vi "Read Control Loop Response Power Analysis (Phase).vi"(8 "error in (no error)":errorcluster, 11 "VISA resource name":refnum<visa-resource-name>) -> (0 "error out":errorcluster, 1 "Gain Crossover Frequency (Hz)":dbl, 2 "Phase Margin (°)":dbl, 3 "VISA resource name out":refnum<visa-resource-name>)   [LabVIEW 2015, in "Agilent 2000 3000 X-Series.lvlib"]
doc: "Returns the phase margin and gain crossover frequency.\n\n<b>Note:</b>\nThis VI is only applicable for 3000T, 3000G, 4000, 6000 X-Series."
uses:
  Agilent 2000 3000 X-Series.lvlib
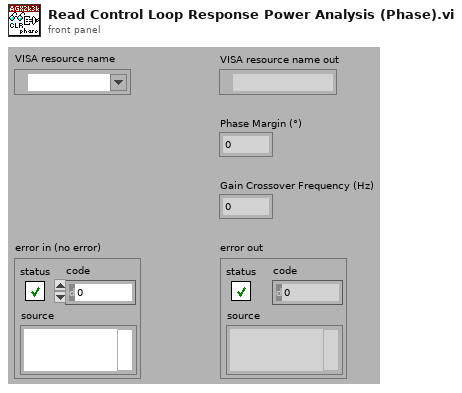
[diagram p1: front panel]
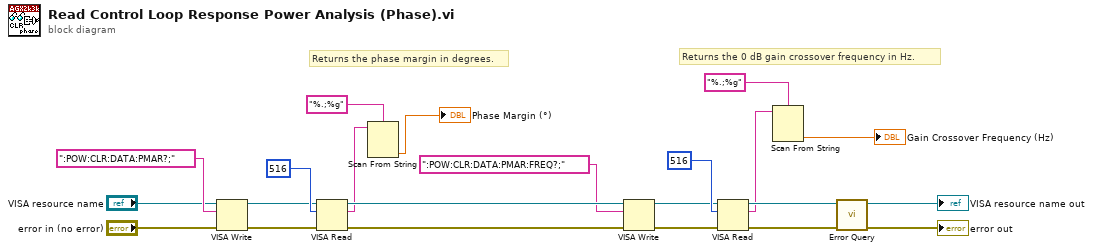
[diagram p0: block diagram]
diagram:
  # "Returns the phase margin in degrees."
  # "Returns the 0 dB gain crossover frequency in Hz."
  n1 = VISA Write(VISA resource name="VISA resource name", write buffer=":POW:CLR:DATA:PMAR?;", error in (no error)="error in (no error)") -> (VISA resource name out=w18:refnum<visa-resource-name>, error out=w17:errorcluster)  [unwired: 1 out]
  n2 = VISA Read(VISA resource name=w18, byte count=516, error in (no error)=w17) -> (VISA resource name out=w13:refnum<visa-resource-name>, read buffer=w7:string, error out=w12:errorcluster)  [unwired: 1 out]
  n3 = Scan From String(format string="%.;%g", input string=w7) -> (output 1=→"Phase Margin (°)":dbl)  [unwired: 3 in, 3 out]
  n4 = VISA Write(VISA resource name=w13, write buffer=":POW:CLR:DATA:PMAR:FREQ?;", error in (no error)=w12) -> (VISA resource name out=w15:refnum<visa-resource-name>, error out=w14:errorcluster)  [unwired: 1 out]
  n5 = VISA Read(VISA resource name=w15, byte count=516, error in (no error)=w14) -> (VISA resource name out=w11:refnum<visa-resource-name>, read buffer=w3:string, error out=w10:errorcluster)  [unwired: 1 out]
  n6 = Scan From String(format string="%.;%g", input string=w3) -> (output 1=→"Gain Crossover Frequency (Hz)":dbl)  [unwired: 3 in, 3 out]
  n7 = call "Error Query.vi"("error in (no error)"=w10, "VISA resource name"=w11) -> ("error out"=→"error out":errorcluster, "VISA resource name out"=→"VISA resource name out":refnum<visa-resource-name>)  [unwired: 6 in, 2 out]
